vi "HexConvertion.vi"(4 "Imaging Protocol":T1, 5 "Laser(V)":dbl[](array[numeric]), 6 "Movement Correction":bool, 7 "AOL_Globals":T3={"Imaging Protocol"=enum."AOL Z-Stack", "Number of POI"=0, "Number of Miniscans"=0, "Number of Trials"=0, "Number of Cycles "=0, "# Averaged Frames"=0, "Laser power (%)"=0, "Pockels (V)"=0.0, "Acquisition Length (sec)"=0.0, "Fill time (us)"=0.0, "POI Dwell time (us)"=0.0, "Miniscan Dwell time per pixel (us)"=0.0, "PMT 1"=0.0, "PMT 2"=0.0, "Back Apperture (mA)"=200.0, "Frame Size"=0, "Center Frequency"=0.0, "Field of View (norm)"=0.0, "DwellTime (us)"=0.0, "Wavelength (nm)"=0.0, "Zoom"=0.0, "AOL Z"=0.0, "AOL Mode"=enum."Raster", "GridXY"=0.0, "GridZ"=0.0, "TriggerPeriod (sec)"=0.0, "Number of Pixels in Miniscan"=0, "Experiment folder path"=path "", "X centre"=0.0, "Y centre"=0.0, "Angle (degrees)"=0.0, "Plane Mode"=0, "Threshold"=[], "Regenerate Chirps"=FALSE, "Rectangle ROI length (pixels)"=0, "Rectangle ROI height (pixels)"=0, "AOD fill"=4900, "StartupDelay"=0, "Samples Wait after Trigger"=5080, "Slip Cycle"=600000, "Add Cycle"=TRUE, "Functional Mode"=enum."Point", "Z Start"=0.0, "Z Stop"=0.0, "# Planes"=0} {"Plane Mode" items=["XY Plane", "XZ Plane", "YZ Plane", "arbitraryplane"]; "Frame Size" items=["100X100"=100, "128X128"=128, "200X200"=200, "256X256"=256, "512X512"=512, "1024x1024"=1024, "2048x2048"=2048]; "Back Apperture (mA)" format="%#.6g"; "Pockels (V)" format="%#.6g"; "PMT 2" format="%#.6g"; "PMT 1" format="%#.6g"; "Angle (degrees)" format="%#.6g"; "POI Dwell time (us)" format="%#.6g"}, 8 "error in (no error)":errorcluster, 11 "Chirp Parameters":T2) -> (0 "error out":errorcluster, 1 "Interrupted":bool, 3 "HexPackets":string[](array[string]))   [LabVIEW 2017]
uses:
  Typedefs/Controls/AOL_Globals.ctl
  Typedefs/Imaging Protocols enum.ctl
  Typedefs/Frame Size.ctl
  Typedefs/AOL modes.ctl
  Typedefs/Plane Mode.ctl
  Typedefs/Functional Mode.ctl
  Typedefs/Chirp_ABCD.ctl
panel:
  in  "aolAmplitudes":T8={"aod1Amplitude"=210.0, "aod2Amplitude"=150.0, "aod3Amplitude"=190.0, "aod4Amplitude"=150.0}
  # "RE-ENTRANT"
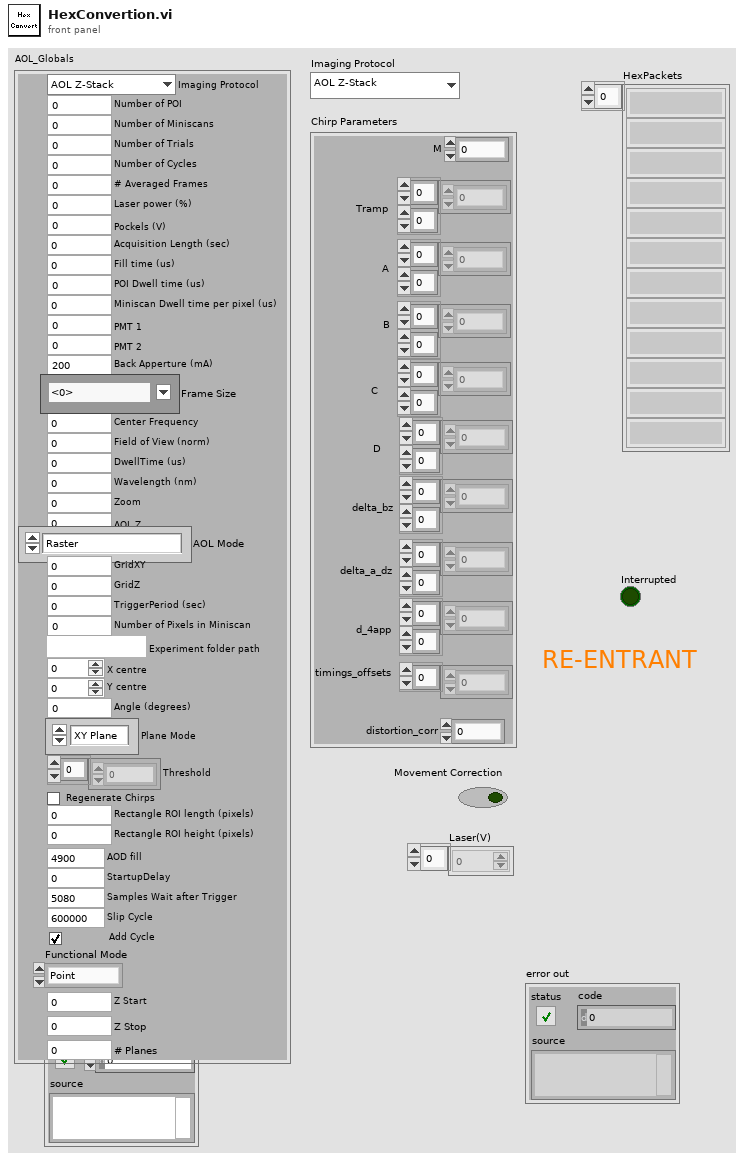
[diagram p1: front panel]
types:
  T1 = typedef "Imaging Protocols enum.ctl" = enum16{"AOL Z-Stack", "Motor Z Stack", "Functional Acquisition", "Single Plane Acquisition", "Volume Acquisition", "Live Imaging", "Live Plane Imaging", "Live Volume Imaging"}
  T2 = typedef "Chirp_ABCD.ctl" = cluster{"M ":dbl, "Tramp":dbl[][], "A":dbl[][], "B":dbl[][], "C":dbl[][], "D":dbl[][], "delta_bz":dbl[][], "delta_a_dz":dbl[][], "d_4app":dbl[][], "timings_offsets":dbl[], "distortion_corr":dbl}
  T3 = typedef "AOL_Globals.ctl" = cluster{"Imaging Protocol":T1, "Number of POI":u16, "Number of Miniscans":u16, "Number of Trials":u16, "Number of Cycles ":u64, "# Averaged Frames":u16, "Laser power (%)":u8, "Pockels (V)":dbl, "Acquisition Length (sec)":dbl, "Fill time (us)":dbl, "POI Dwell time (us)":dbl, "Miniscan Dwell time per pixel (us)":dbl, "PMT 1":dbl, "PMT 2":dbl, "Back Apperture (mA)":dbl, "Frame Size":T4, "Center Frequency":dbl, "Field of View (norm)":dbl, "DwellTime (us)":dbl, "Wavelength (nm)":dbl, "Zoom":dbl, "AOL Z":dbl, "AOL Mode":T5, "GridXY":dbl, "GridZ":dbl, "TriggerPeriod (sec)":dbl, "Number of Pixels in Miniscan":u16, "Experiment folder path":path, "X centre":dbl, "Y centre":dbl, "Angle (degrees)":dbl, "Plane Mode":T6, "Threshold":u16[], "Regenerate Chirps":bool, "Rectangle ROI length (pixels)":u16, "Rectangle ROI height (pixels)":u16, "AOD fill":u16, "StartupDelay":i32, "Samples Wait after Trigger":u16, "Slip Cycle":u32, "Add Cycle":bool, "Functional Mode":T7, "Z Start":dbl, "Z Stop":dbl, "# Planes":i32}
  T4 = typedef "Frame Size.ctl" = u16
  T5 = typedef "AOL modes.ctl" = enum16{"Raster", "Structural", "Pointing", "Mini Scan", "Alignment"}
  T6 = typedef "Plane Mode.ctl" = u16
  T7 = typedef "Functional Mode.ctl" = enum16{"Point", "Line", "Patch", "Plane", "Volume"}
  T8 = cluster{"aod1Amplitude":dbl, "aod2Amplitude":dbl, "aod3Amplitude":dbl, "aod4Amplitude":dbl}
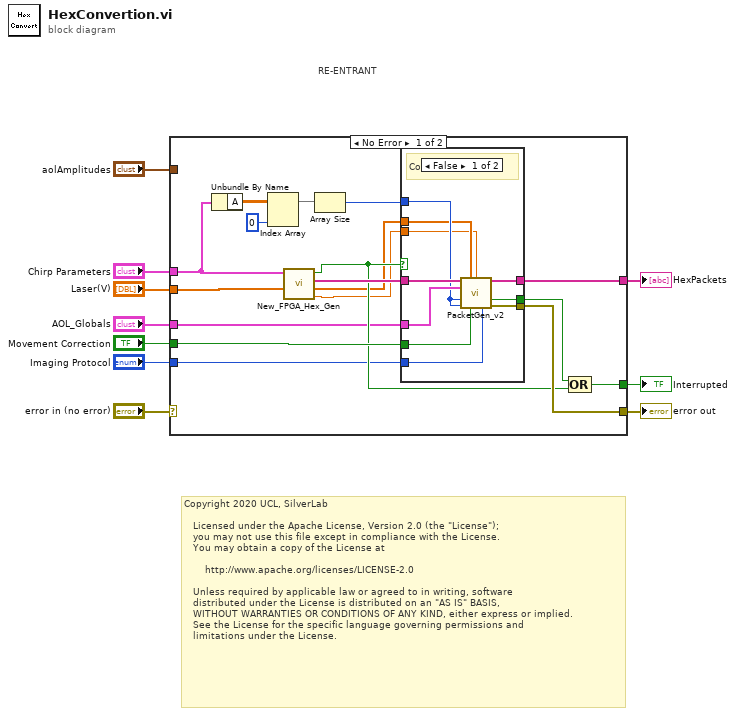
[diagram p0: block diagram]
diagram:
  # "Copyright 2020 UCL, SilverLab\n \n   Licensed under the Apache License, Version 2.0 (the \"License\");\n   you may not use this file except in compliance with the License.\n   You may obtain a copy of the License at\n \n       http://www.apache.org/licenses/LICENSE-2.0\n \n   Unless required by applicable law or agreed to in writing, software\n   distributed under the License is distributed on an \"AS IS\" BASIS,\n   WITHOUT WARRANTIES OR CONDITIONS OF ANY KIND, either express or implied.\n   See the License for the specific language governing permissions and\n   limitations under the License."
  # "RE-ENTRANT"
  n1 = case shown="No Error" "error in (no error)" {
    selector: "error in (no error)" -> [_ w38]
    tunnel: [w23 w38] -> w9
    tunnel: "aolAmplitudes" -> [_ _]
    tunnel: "AOL_Globals" -> [w13 _]
    tunnel: [w27 _] -> w6
    tunnel: "Chirp Parameters" -> [w15 _]
    tunnel: [w20 _] -> w4
    tunnel: "Movement Correction" -> [w19 _]
    tunnel: "Imaging Protocol" -> [w16 _]
    tunnel: "Laser(V)" -> [w14 _]
    frame No Error {
      n2 = Unbundle By Name(w15) -> ("A"=w26:dbl[][])
      n3 = Index Array(array=w26, index (col)=0 ("disabled index (col)")) -> (element=w25:dbl[])  [unwired: 1 in]
      n4 = call "New_FPGA_Hex_Gen.vi"("Laser(V)"=w14, "Chirp Parameters"=w15) -> ("distortion_corr"=w11:dbl, "timings_offsets"=w12:dbl[], "HEX Array"=w22:string[], "Interrupted"=w18:bool)  [unwired: 6 in]
      n5 = Array Size(array=w25) -> (size(s)=w17:i32)
      n6 = case shown="False" w18 {
        tunnel: w13 -> [w37 _]
        tunnel: [w36 _] -> w27
        tunnel: w17 -> [w31 _]
        tunnel: [w35 _] -> w23
        tunnel: w22 -> [w34 _]
        tunnel: [w33 _] -> w21
        tunnel: w19 -> [w32 _]
        tunnel: w16 -> [w30 _]
        tunnel: w12 -> [w29 _]
        tunnel: w11 -> [w28 _]
        frame False {
          # "Continue"
          n7 = call "PacketGen_v2.vi"("Hex Array"=w34, "timings_offsets"=w29, "distortion_corr"=w28, "AOL_Globals"=w37, "Ny"=w31, "Nx"=w31, "Movement Correction"=w32, "Imaging Protocol"=w30) -> ("HexPackets"=w36:string[], "Interrupted"=w33:bool, "error out"=w35:errorcluster)  [unwired: 4 in, 1 out]
        }
        frame True {
          # "Interrupted"
        }
      }
      n8 = Compound Arithmetic op=OR(w21, w18) -> (w20:bool)
    }
    frame Error {
    }
  }
  "error out" <- w9
  "HexPackets" <- w6
  "Interrupted" <- w4
